vi "Constants.vi"() -> ()   [LabVIEW 2026, in "Runtime Configuration Support Inline Async Example Custom Device Shared.lvlib"]
doc: "Use this Global VI to access the GUIDs assigned to the page resources of the Custom Device."
uses:
  Runtime Configuration Support Inline Async Example Custom Device Shared.lvlib
panel:
  in  "Tab Control":enum32{"GUIDs", "Constants", "Properties"}(tab)
  in  "Runtime Configuration Support Inline Async Example Custom Device":string="c67b4315-6b50-49ec-9d9f-ed5924ef5663"
  in  "Compiled.Settings":string="Compiled.Settings"
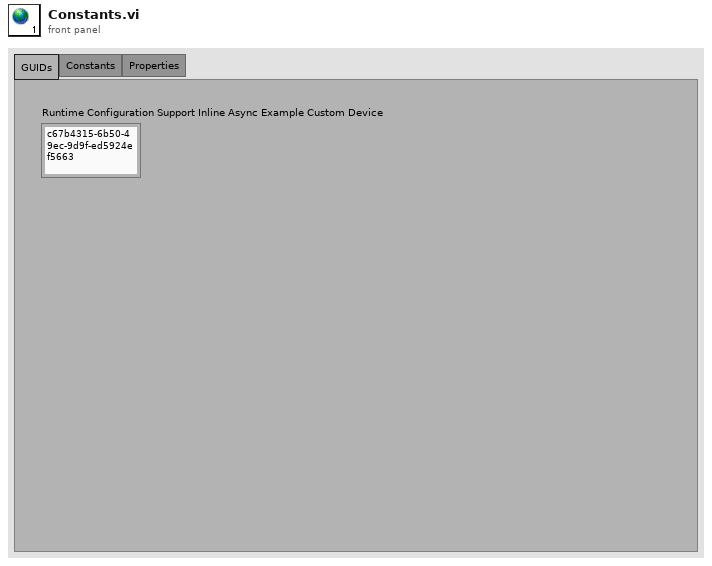
[diagram p1: front panel]
diagram:
